vi "svl_Filter Coefficients [Order 2].vi"(11 "dt":dbl) -> (2 "filter coefficients":cluster{"beta":dbl, "gamma":dbl, "alpha":dbl} {"alpha" format="%.2f"; "gamma" format="%.2f"; "beta" format="%.2f"})   [LabVIEW 2017, in "SoundVib_Integration.lvlib"]
uses:
  <vilib>/addons/Sound and Vibration/svt_Integration/SoundVib_Integration.lvlib
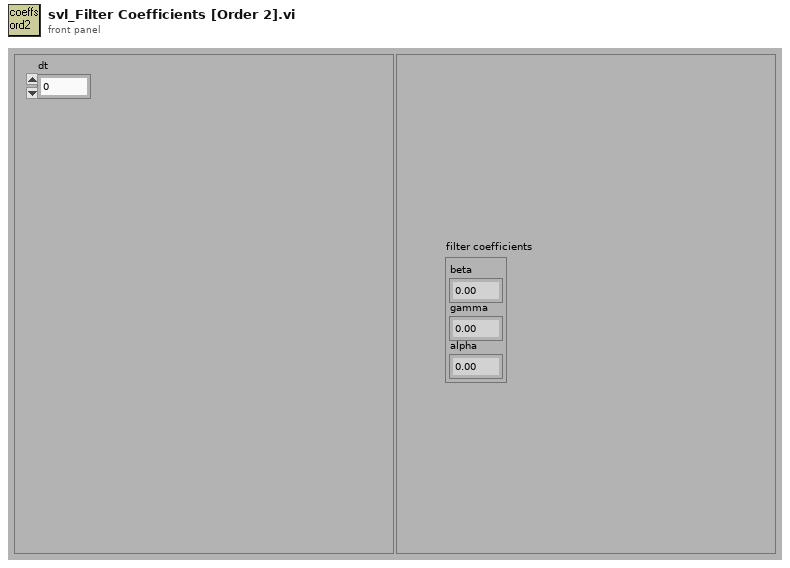
[diagram p1: front panel]
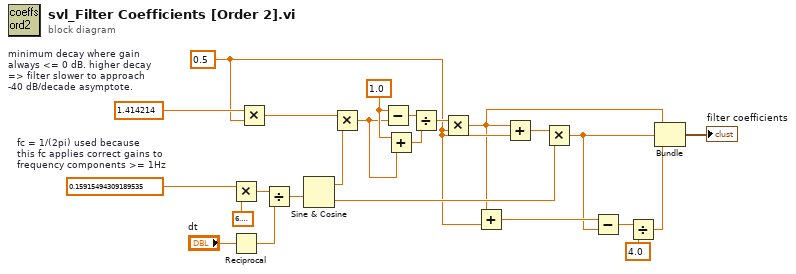
[diagram p0: block diagram]
diagram:
  w6 = 0.5 ("y")
  w16 = 1.0 ("x")
  w22 = 1.414214  # minimum decay where gain  always <= 0 dB. higher decay => filter slower to approach  -40 dB/decade asymptote.
  w23 = 0.15915494309189535  # fc = 1/(2pi) used because  this fc applies correct gains to  frequency components >= 1Hz
  n1 = Multiply(x=w23, y=6.283185307179586) -> (x*y=w20:dbl)
  n2 = Reciprocal(x="dt") -> (1/x=w5:dbl)
  n3 = Multiply(x=w22, y=w6) -> (x*y=w18:dbl)
  n4 = Divide(x=w20, y=w5) -> (x/y=w19:dbl)
  n5 = Sine & Cosine(0:w19) -> (1:w17:dbl, 2:w10:dbl)
  n6 = Multiply(x=w18, y=w17) -> (x*y=w15:dbl)
  n7 = Subtract(x=w16, y=w15) -> (x-y=w14:dbl)
  n8 = Add(x=w16, y=w15) -> (x+y=w13:dbl)
  n9 = Divide(x=w14, y=w13) -> (x/y=w12:dbl)
  n10 = Multiply(x=w12, y=w6) -> (x*y=w3:dbl)
  n11 = Add(x=w3, y=w6) -> (x+y=w9:dbl)
  n12 = Add(x=w3, y=w6) -> (x+y=w11:dbl)
  n13 = Multiply(x=w11, y=w10) -> (x*y=w4:dbl)
  n14 = Subtract(x=w9, y=w4) -> (x-y=w8:dbl)
  n15 = Divide(x=w8, y=4.0) -> (x/y=w24:dbl)
  n16 = Bundle(w3, w4, w24) -> (→"filter coefficients":cluster{dbl, dbl, dbl})  [unwired: 1 in]
